vi "Add_filename_to_err_message.vi"(1 "error in (no error)":errorcluster, 2 "Path":path) -> (0 "error out":errorcluster)   [LabVIEW 2010]
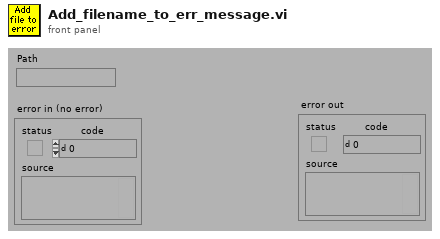
[diagram p1: front panel]
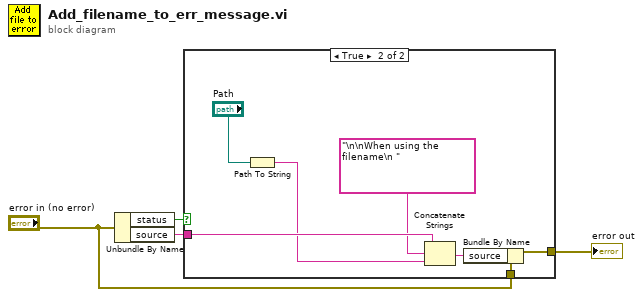
[diagram p0: block diagram]
diagram:
  n1 = Unbundle By Name("error in (no error)") -> ("status"=w1:bool, "source"=w4:string)
  n2 = case shown="True" w1 {
    tunnel: w4 -> [_ w11]
    tunnel: [w5 w9] -> w3
    tunnel: "error in (no error)" -> [w5 w8]
    frame False {
    }
    frame True {
      n3 = Path To String(path="Path") -> (string=w6:string)
      n4 = Concatenate Strings(w11, "\n\nWhen using the filename\n ", w6) -> (w12:string)
      n5 = Bundle By Name(cluster=w8, "source"=w12) -> (w9:errorcluster)
    }
  }
  "error out" <- w3
